vi "Teleop.vi"(0 "Call Context":T2, 1 "Match Info":T1={"Autonomous Elapsed Seconds"=0.0, "TeleOp Elapsed Seconds"=0.0, "Disabled Elapsed Seconds"=0.0, "Visited Autonomous"=FALSE, "Visited TeleOp"=FALSE, "Visited Disabled"=FALSE, "Autonomous Settings"={"Autonomous Style"=enum."Independent", "VI Refnum"=refnum}}) -> ()   [LabVIEW 2011]
doc: "This VI is called for each TeleOp packet received from the DS where the robot is not disabled. It is often used to read from the joysticks and update I/O or to update setpoints for timed control loops. It should complete and return within 20 milliseconds or it may miss DS packets."
uses:
  <vilib>/Rock Robotics/WPI/DriverStation/WPI_DriverStationDerivedRobotMode.ctl
  <vilib>/Rock Robotics/WPI/DriverStation/WPI_DriverStationMatch Info.ctl
  Robot Global Data.vi
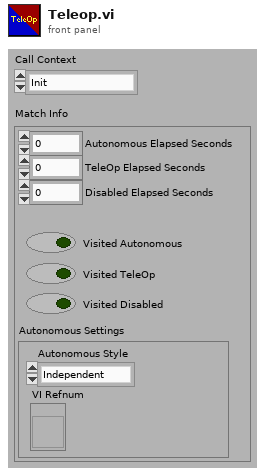
[diagram p1: front panel]
types:
  T1 = typedef "WPI_DriverStationMatch Info.ctl" = cluster{"Autonomous Elapsed Seconds":dbl, "TeleOp Elapsed Seconds":dbl, "Disabled Elapsed Seconds":dbl, "Visited Autonomous":bool, "Visited TeleOp":bool, "Visited Disabled":bool, "Autonomous Settings":cluster{"Autonomous Style":enum16{"Iterative", "Independent"}, "VI Refnum":refnum<vi>}}
  T2 = typedef "WPI_DriverStationDerivedRobotMode.ctl" = enum16{"Init", "Execute", "Stop"}
  T3 = typedef "WPI_JoystickDevRef.ctl" = cluster{"Device":T4}
  T4 = typedef "WPI_JoystickDeviceEnum.ctl" = enum16{"USB 1", "USB 2", "USB 3", "USB 4", "Kinect 1", "Kinect 2"}
  T5 = typedef "WPI_JoystickButtonState.ctl" = cluster{"Button 1":bool, "Button 2":bool, "Button 3":bool, "Button 4":bool, "Button 5":bool, "Button 6":bool, "Button 7":bool, "Button 8":bool, "Button 9":bool, "Button 10":bool, "Button 11":bool, "Button 12":bool}
  T6 = cluster{"axis 1 (x)":dbl, "axis 2 (y)":dbl, "axis 3 (throttle)":dbl, "axis 4":dbl, "axis 5":dbl, "axis 6":dbl}
  T7 = typedef "WPI_RobotDriveDevRef.ctl" = cluster{"DevStatus":errorcluster, "Motors[]":T8[], "Square Inputs":bool, "Max Output":dbl, "Isochronous":bool}
  T8 = typedef "WPI_MotorControlDeviceRef.ctl" = cluster{"DeviceStatus":errorcluster, "Type":enum16{"PWM", "CAN"}, "PWM":cluster{"Digital Module":T9, "PWM Channel":T10, "DeadBand":T11}, "CAN":cluster{"Device Number":u8, "Control Mode":T12, "Semaphore":T13, "Max Vout":dbl}, "Invert":bool, "TransformRef":T14, "InvTransformRef":T14}
  T9 = typedef "FPGA_TypedefDigitalModule.ctl" = enum16{"Digital Module 1", "Digital Module 2"}
  T10 = typedef "FPGA_DIOPWMChannel.ctl" = enum8{"PWM 1", "PWM 2", "PWM 3", "PWM 4", "PWM 5", "PWM 6", "PWM 7", "PWM 8", "PWM 9", "PWM 10", "Invalid"}
  T11 = typedef "WPI_PWMDeadband.ctl" = cluster{"Name":string, "maxPositivePwm":i32, "minPositivePwm":i32, "centerPwm":i32, "maxNegativePwm":i32, "minNegativePwm":i32, "angularRange":u16}
  T12 = typedef "WPI_CANJaguar_ControlMode.ctl" = enum8{"Percent VBus", "Current", "Speed", "Position", "Voltage"}
  T13 = typedef "Semaphore RefNum" = refnum<k1>
  T14 = typedef "WPI_PWMTransform_ConPane.ctl" = refnum<vi>
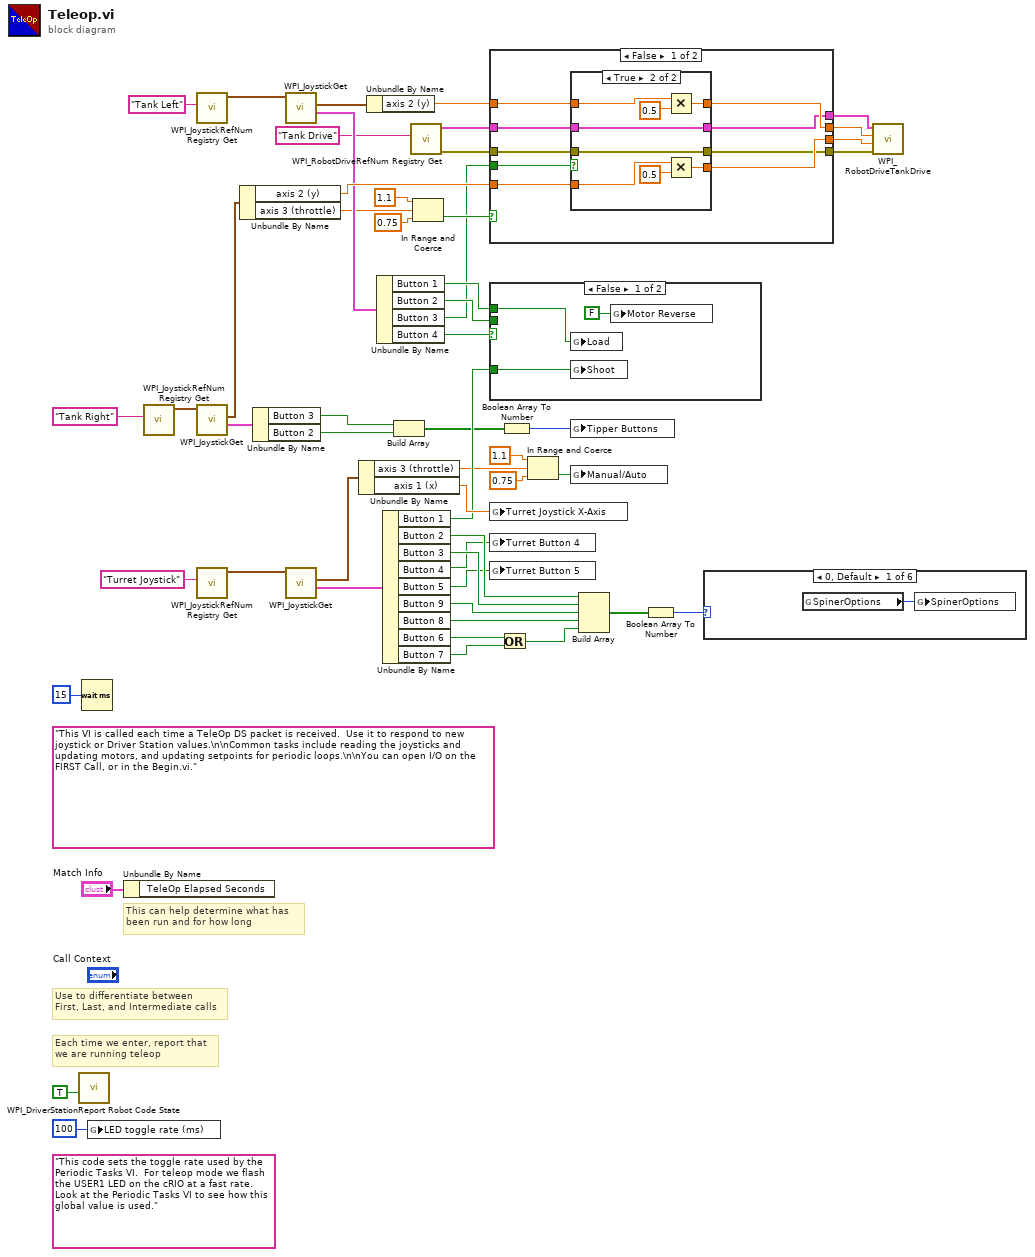
[diagram p0: block diagram]
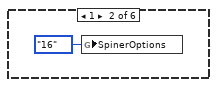
[diagram p2: hidden frame]
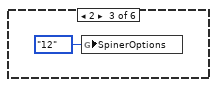
[diagram p3: hidden frame]
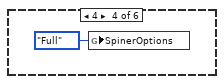
[diagram p4: hidden frame]
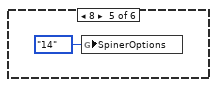
[diagram p5: hidden frame]
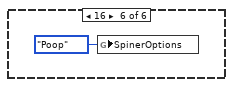
[diagram p6: hidden frame]
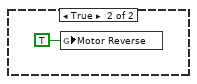
[diagram p7: hidden frame]
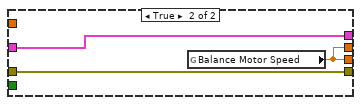
[diagram p9: hidden frame]
diagram:
  (unwired) "This code sets the toggle rate used by the Periodic Tasks VI.  For teleop mode we flash the USER1 LED on the cRIO at a fast rate.  Look at the Periodic Tasks VI to see how this global value is used."
  (unwired) "This VI is called each time a TeleOp DS packet is received.  Use it to respond to new joystick or Driver Station values.\n\nCommon tasks include reading the joysticks and updating motors, and updating setpoints for periodic loops.\n\nYou can open I/O on the FIRST Call, or in the Begin.vi."
  # "Each time we enter, report that\nwe are running teleop"
  # "Use to differentiate between\nFirst, Last, and Intermediate calls"
  # "This can help determine what has\nbeen run and for how long"
  n1 = call <vilib>:"WPI_DriverStationReport Robot Code State.vi"("TeleOp"=TRUE ("Autonomous")) -> ()  [unwired: 10 in, 1 out]
  n2 = Wait (ms)(milliseconds to wait=u32 15) -> ()  [unwired: 1 out]
  n3 = global write "Robot Global Data.vi" "LED toggle rate (ms)"(u32 100 ("LED ms toggle rate")) -> ()
  n4 = Unbundle By Name("Match Info") -> ()  [unwired: 1 out]
  n5 = call <vilib>:"WPI_JoystickRefNum Registry Get.vi"("refnum name"="Tank Right") -> ("JoystickDevRef"=w48:T3)  [unwired: 9 in, 1 out]
  n6 = call <vilib>:"WPI_JoystickRefNum Registry Get.vi"("refnum name"="Tank Left") -> ("JoystickDevRef"=w50:T3)  [unwired: 9 in, 1 out]
  n7 = call <vilib>:"WPI_JoystickGet.vi"("JoystickDevRef"=w48) -> ("Buttons"=w8:T5, "Axes"=w43:T6)  [unwired: 1 in, 4 out]
  n8 = call <vilib>:"WPI_JoystickRefNum Registry Get.vi"("refnum name"="Turret Joystick") -> ("JoystickDevRef"=w35:T3)  [unwired: 1 in, 9 out]
  n9 = Unbundle By Name(w43) -> ("axis 2 (y)"=w44:dbl, "axis 3 (throttle)"=w31:dbl)
  n10 = Unbundle By Name(w8) -> ("Button 3"=w6:bool, "Button 2"=w7:bool)
  n11 = call <vilib>:"WPI_JoystickGet.vi"("JoystickDevRef"=w50) -> ("Buttons"=w41:T5, "Axes"=w42:T6)  [unwired: 1 in, 4 out]
  n12 = call <vilib>:"WPI_JoystickGet.vi"("JoystickDevRef"=w35) -> ("Buttons"=w34:T5, "Axes"=w37:T6)  [unwired: 1 in, 4 out]
  n13 = Unbundle By Name(w37) -> ("axis 3 (throttle)"=w20:dbl, "axis 1 (x)"=w30:dbl)
  n14 = Unbundle By Name(w42) -> ("axis 2 (y)"=w45:dbl)
  n15 = Unbundle By Name(w41) -> ("Button 1"=w25:bool, "Button 2"=w24:bool, "Button 3"=w13:bool, "Button 4"=w19:bool)
  n16 = Unbundle By Name(w34) -> ("Button 1"=w26:bool, "Button 2"=w18:bool, "Button 3"=w17:bool, "Button 4"=w12:bool, "Button 5"=w11:bool, "Button 9"=w14:bool, "Button 8"=w4:bool, "Button 6"=w2:bool, "Button 7"=w1:bool)
  n17 = Build Array(w6, w7) -> (w9:bool[])
  n18 = call <vilib>:"WPI_RobotDriveRefNum Registry Get.vi"("refnum name"="Tank Drive") -> ("error out"=w46:errorcluster, "RobotDriveDevRef"=w47:T7)  [unwired: 9 in]
  n19 = In Range and Coerce(upper limit=1.1, x=w31, lower limit=0.75) -> (In Range?=w21:bool)  [unwired: 1 out]
  n20 = case shown="False" w21 {
    tunnel: w47 -> [w63 w76]
    tunnel: w46 -> [w62 w77]
    tunnel: w45 -> [w60 _]
    tunnel: w44 -> [w61 _]
    tunnel: [w58 w76] -> w28
    tunnel: [w57 w78] -> w22
    tunnel: [w59 w78] -> w23
    tunnel: [w56 w77] -> w27
    tunnel: w13 -> [w55 _]
    frame False {
      n21 = case shown="True" w55 {
        tunnel: w63 -> [w65 w70]
        tunnel: w62 -> [w64 w68]
        tunnel: w61 -> [w67 w71]
        tunnel: w60 -> [w66 w75]
        tunnel: [w66 w73] -> w59
        tunnel: [w65 w70] -> w58
        tunnel: [w67 w69] -> w57
        tunnel: [w64 w68] -> w56
        frame False {
        }
        frame True {
          n22 = Multiply(x=w75, y=0.5) -> (x*y=w73:dbl)
          n23 = Multiply(x=w71, y=0.5) -> (x*y=w69:dbl)
        }
      }
    }
    frame True {
      n24 = global read "Robot Global Data.vi" "Balance Motor Speed"() -> (w78:dbl)
    }
  }
  n25 = case shown="False" w19 {
    tunnel: w26 -> [w81 _]
    tunnel: w25 -> [w80 _]
    tunnel: w24 -> [_ _]
    frame False {
      n26 = global write "Robot Global Data.vi" "Load"(w80) -> ()
      n27 = global write "Robot Global Data.vi" "Shoot"(w81) -> ()
      n28 = global write "Robot Global Data.vi" "Motor Reverse"(FALSE ("Motor Reverse")) -> ()
    }
    frame True {
      n29 = global write "Robot Global Data.vi" "Motor Reverse"(TRUE ("Motor Reverse")) -> ()
    }
  }
  n30 = global write "Robot Global Data.vi" "Turret Joystick X-Axis"(w30) -> ()
  n31 = global write "Robot Global Data.vi" "Turret Button 4"(w12) -> ()
  n32 = global write "Robot Global Data.vi" "Turret Button 5"(w11) -> ()
  n33 = Or(x=w2, y=w1) -> (x .or. y?=w3:bool)
  n34 = Boolean Array To Number(Boolean array=w9) -> (number=w10:u32)
  n35 = In Range and Coerce(upper limit=1.1, x=w20, lower limit=0.75) -> (In Range?=w29:bool)  [unwired: 1 out]
  n36 = global write "Robot Global Data.vi" "Tipper Buttons"(w10) -> ()
  n37 = global write "Robot Global Data.vi" "Manual/Auto"(w29) -> ()
  n38 = Build Array(w18, w17, w14, w4, w3) -> (w16:bool[])
  n39 = Boolean Array To Number(Boolean array=w16) -> (number=w15:u32)
  n40 = case shown="0, Default" w15 {
    frame 0, Default {
      n41 = global read "Robot Global Data.vi" "SpinerOptions"() -> (w83:enum16{"Full", "16", "14", "12", "Poop"})
      n42 = global write "Robot Global Data.vi" "SpinerOptions"(w83) -> ()
    }
    frame 1 {
      n43 = global write "Robot Global Data.vi" "SpinerOptions"(enum16{"Full", "16", "14", "12", "Poop"}."16" ("SpinerOptions")) -> ()
    }
    frame 2 {
      n44 = global write "Robot Global Data.vi" "SpinerOptions"(enum16{"Full", "16", "14", "12", "Poop"}."12" ("SpinerOptions")) -> ()
    }
    frame 4 {
      n45 = global write "Robot Global Data.vi" "SpinerOptions"(enum16{"Full", "16", "14", "12", "Poop"}."Full" ("SpinerOptions")) -> ()
    }
    frame 8 {
      n46 = global write "Robot Global Data.vi" "SpinerOptions"(enum16{"Full", "16", "14", "12", "Poop"}."14" ("SpinerOptions")) -> ()
    }
    frame 16 {
      n47 = global write "Robot Global Data.vi" "SpinerOptions"(enum16{"Full", "16", "14", "12", "Poop"}."Poop" ("SpinerOptions")) -> ()
    }
  }
  n48 = call <vilib>:"WPI_RobotDriveTankDrive.vi"("error in (no error)"=w27, "Right axis value"=w22, "Left axis value"=w23, "RobotDriveDevRef"=w28) -> ()  [unwired: 6 in, 2 out]
